vi "Perform Action.vi"(8 "error in":errorcluster, 10 "Input":variant, 11 "Thermometer DAQmx RTD Cont CFG in":refnum<class "Thermometer DAQmx RTD Cont CFG.lvclass">) -> (0 "error out":errorcluster, 2 "Output":variant, 3 "Thermometer DAQmx RTD Cont CFG out":refnum<class "Thermometer DAQmx RTD Cont CFG.lvclass">)   [LabVIEW 2024, in "Thermometer DAQmx RTD Cont CFG.lvclass"]
uses:
  Thermometer DAQmx RTD Cont CFG.lvclass
  D:/git/HAL/HAL/Devices/DAQmx/DAQmx Base CFG/DAQmx Base CFG.lvclass
  DAQmx Base CFG/DAQmx Base CFG.lvclass/DAQmx Base CFG.ctl
  Thermometer DAQmx RTD Cont CFG.lvclass/Thermometer DAQmx RTD Cont CFG.ctl
  <vilib>/DAQmx/read.llb/DAQmx Read (Analog 2D DBL NChan NSamp).vi
  <vilib>/DAQmx/miscellaneous.llb/DAQmx Fill In Error Info.vi
  DAQmx Base CFG/DAQmx Base CFG.lvclass
  Buffers/BufferLastReadingsDBL/BufferLastReadsDBL.lvclass
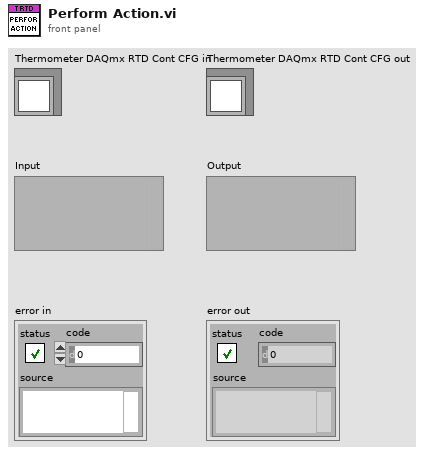
[diagram p1: front panel]
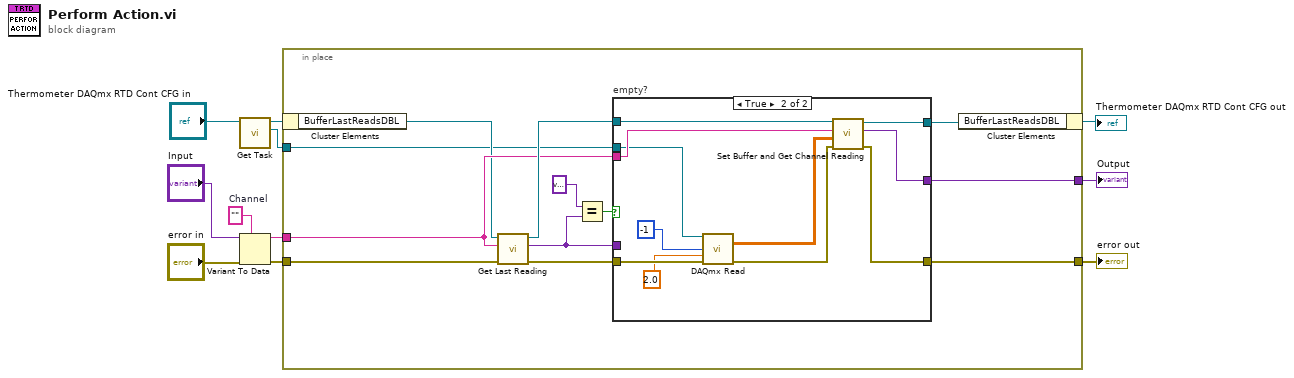
[diagram p0: block diagram]
diagram:
  w7 = ""  # Channel
  n1 = call "Get Task.vi"("DAQmx Base CFG in"="Thermometer DAQmx RTD Cont CFG in") -> ("Task"=w4:refnum<k21>, "DAQmx Base CFG out"=w2:refnum<class "Thermometer DAQmx RTD Cont CFG.lvclass">)  [unwired: 9 in]
  n2 = Variant To Data(error in="error in", type=w7, Variant="Input") -> (data=w5:string, error out=w6:errorcluster)
  n3 = in-place {
    in-place-border: [w21] -> w9
    in-place-border: [w20] -> w8
    in-place-border: w6 -> [w19]
    in-place-border: w5 -> [w18]
    in-place-border: w4 -> [w13]
    n4 = in-place-cluster #1(w2) -> ("BufferLastReadsDBL"=w14:refnum<class "BufferLastReadsDBL.lvclass">)
    n5 = call "Get Last Reading.vi"("error in"=w19, "Channel"=w18, "BufferLastReadingsDBL in"=w14) -> ("error out"=w22:errorcluster, "Last Read"=w15:variant, "BufferLastReadingsDBL out"=w23:refnum<class "BufferLastReadsDBL.lvclass">)  [unwired: 6 in]
    n6 = Equal?(x=variant, y=w15) -> (x = y?=w17:bool)
    n7 = case "empty?" shown="True" w17 {
      tunnel: w23 -> [w25 w27]
      tunnel: w22 -> [w24 w34]
      tunnel: [w24 w36] -> w21
      tunnel: [w26 w31] -> w20
      tunnel: [w25 w35] -> w12
      tunnel: w15 -> [w26 _]
      tunnel: w18 -> [_ w32]
      tunnel: w13 -> [_ w28]
      frame False {
      }
      frame True {
        n8 = call-poly <vilib>:"DAQmx Read.vi"("task/channels in"=w28, "number of samples per channel"=-1, "timeout"=2.0, "error in"=w34) -> ("data"=w33:dbl[][], "error out"=w37:errorcluster)  [unwired: 9 in, 1 out]
        n9 = call "Set Buffer and Get Channel Reading.vi"("error in"=w37, "Readings"=w33, "Channel Ident"=w32, "BufferLastReadingsDBL in"=w27) -> ("error out"=w36:errorcluster, "Last Read"=w31:variant, "BufferLastReadingsDBL out"=w35:refnum<class "BufferLastReadsDBL.lvclass">)  [unwired: 5 in]
      }
    }
    n10 = in-place-cluster #1("BufferLastReadsDBL"=w12) -> (→"Thermometer DAQmx RTD Cont CFG out":refnum<class "Thermometer DAQmx RTD Cont CFG.lvclass">)
  }
  "error out" <- w9
  "Output" <- w8
